vi "TurningSailSuggestion.vi"(6 "Old Suggested Sail Setpoints":T1 {"MainSailSuggestion" min=0.0 max=1.0; "JibSailSuggestion" min=0.0 max=1.0}, 9 "RelativeWindAngle":dbl, 10 "DesiredHeading":dbl, 11 "RobotHeading":dbl) -> (3 "Suggested Sail Setpoints":T1 {"MainSailSuggestion" min=0.0 max=1.0; "JibSailSuggestion" min=0.0 max=1.0})   [LabVIEW 2012]
doc: "Sets the sails in such a way as to help the boat turn in the desired direction. Turning upwind, for example, would involve overpowering the main and underpowering the jib.\n\nWhen exactly this setting should be used is unclear, it probably shouldn't be used for small turns until much testing has been done to make sure it doesn't interfere with regular sail operations. At the moment it seems reasonable to use this to help the boat turn large angles at low speeds. At higher speeds the rudder should be effective to turn the boat.\n\nSuggestion: ONLY calculate how to set the sails to help turn the boat in this VI, use the arbiter to decide when to use the sails to turn.\n\nEric Schneider and Bonnie Ishiguro, Jan. 2014"
uses:
  Data/TypeDefs/Sail Set Suggestions.ctl
panel:
  # "Sets the sails in such a way as to help the boat turn\nin the desired direction. Turning upwind, for example,\nwould involve overpowering the main and underpowering\nthe jib.\n\nWhen exactly this setting should be used is unclear, it\nprobably shouldn't be used for small turns until much testing\nhas been done to make sure it doesn't interfere with regular\nsail operations. At the moment it seems reasonable to use\nthis to help the boat turn large angles at low speeds. At higher\nspeeds the rudder should be effective to turn the boat.\n\nSuggestion: ONLY calculate how to set the sails to help\nturn the boat in this VI, use the arbiter to decide when\nto use the sails to turn."
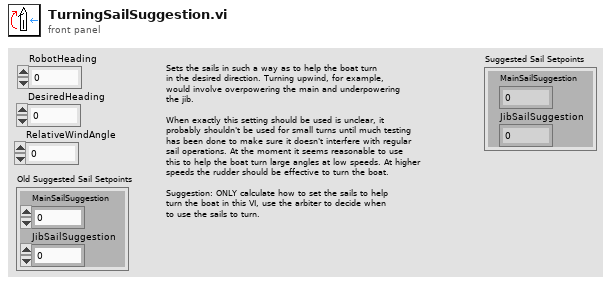
[diagram p1: front panel]
types:
  T1 = typedef "Sail Set Suggestions.ctl" = cluster{"MainSailSuggestion":dbl, "JibSailSuggestion":dbl}
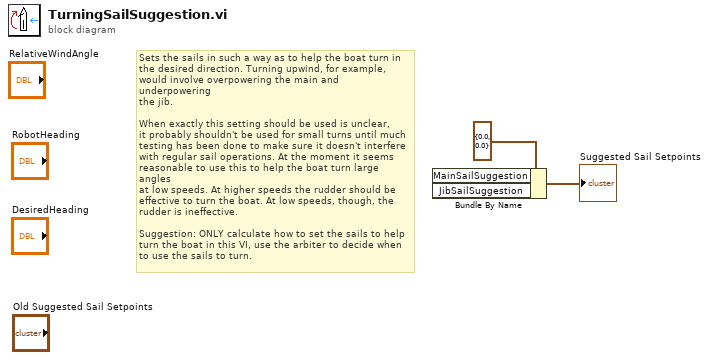
[diagram p0: block diagram]
diagram:
  # "Sets the sails in such a way as to help the boat turn in\nthe desired direction. Turning upwind, for example,\nwould involve overpowering the main and underpowering\nthe jib.\n\nWhen exactly this setting should be used is unclear,\nit probably shouldn't be used for small turns until much\ntesting has been done to make sure it doesn't interfere\nwith regular sail operations. At the moment it seems\nreasonable to use this to help the boat turn large angles\nat low speeds. At higher speeds the rudder should be\neffective to turn the boat. At low speeds, though, the\nrudder is ineffective.\n\nSuggestion: ONLY calculate how to set the sails to help\nturn the boat in this VI, use the arbiter to decide when\nto use the sails to turn."
  n1 = Bundle By Name(cluster=T1 {"MainSailSuggestion"=0.0, "JibSailSuggestion"=0.0} ("output cluster")) -> (→"Suggested Sail Setpoints":T1)  [unwired: 2 in]
